vi "ALTS-2015 _LV2GBL Mode.vi"(7 "Options":T1=enum."Read Mode", 8 "Error In":errorcluster, 10 "Auto Mode?":bool) -> (0 "Error Out":errorcluster, 2 "Auto mode?":bool)   [LabVIEW 2013]
doc: "There are two modes\neither Automatic or Manual\nIf the Boolean is true then the mode is Automatic"
uses:
  Controls/ALTS-2015 Mode Cases.ctl
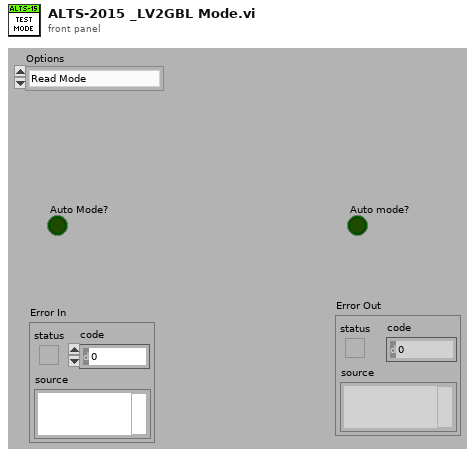
[diagram p1: front panel]
types:
  T1 = typedef "ALTS-2015 Mode Cases.ctl" = enum16{"Set Mode", "Read Mode"}
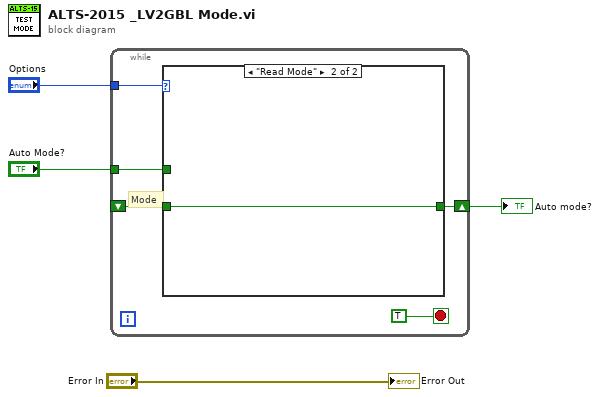
[diagram p0: block diagram]
diagram:
  n1 = while {
    tunnel: "Options" -> [w8]
    tunnel: "Auto Mode?" -> [w7]
    shift-right: [w5] -> w1
    shift-left: _ -> [w6]
    stop <- TRUE stop-if-true
    # "Mode"
    n2 = case shown="\"Read Mode\"" w8 {
      tunnel: w7 -> [w10 _]
      tunnel: w6 -> [_ w11]
      tunnel: [w10 w11] -> w5
      frame "Set Mode" {
      }
      frame "Read Mode" {
      }
    }
  }
  "Auto mode?" <- w1
  "Error Out" <- "Error In"
